vi "15_NOV_UPDATE_2.vi"() -> ()   [LabVIEW 2020]
uses:
  <instrlib>/Agilent B2900 Series/Agilent B2900 Series.lvlib
panel:
  out "Waveform Chart 2":dbl(graph)
  in  "Save data":bool
  in  "File_name":path=path "saved_data"
  out "Y -axis":string
  out "X -axis":string
  out "String":string
  out "SCPI Command":string
  out "?":bool
  in  "Time interval between iterations (seconds)":dbl
  out "?":cluster{"X":dbl[], "Y":dbl[]}[](graph)
  out "Waveform Chart":dbl(graph)
  out "Measured Output Value":dbl
  in  "SELECT DEVICE":refnum<visa-resource-name>="USB0::0x0957::0x8E18::MY51140695::INSTR"
  out "Resolution":dbl format="%#_6f"
  out "Instantaneous Input Value":dbl format="%#_6f"
  in  "Final Value":dbl
  in  "Initial Value":dbl
  in  "Steps":dbl
  in  "Measure (OUTPUT)":enum16{"Voltage", "Current"}(ring)
  in  "Source":enum16{"Voltage", "Current"}(ring)
  in  "Channel":u16(ring) items=["1", "2"]
  # "1. Include file extension .txt after filename while saving\n\n2. Give unique filename to avoid overwriting data."
  # "(INPUT)"
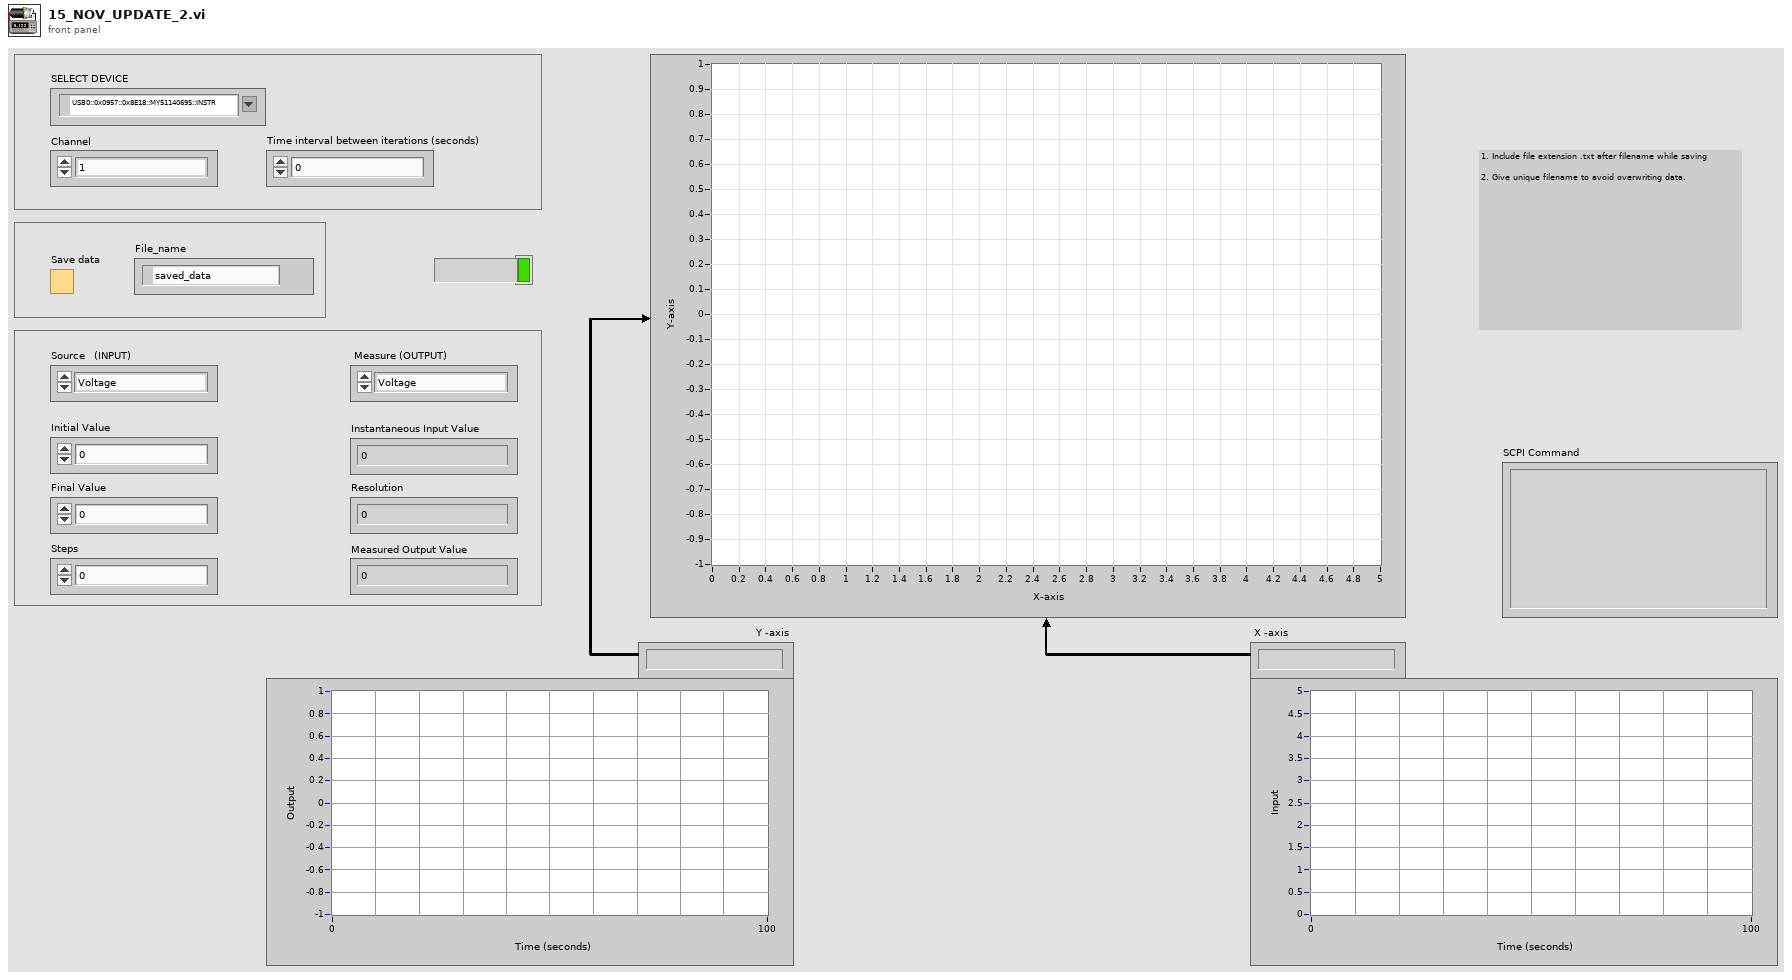
[diagram p1: front panel]
types:
  T1 = enum16{"open", "replace", "create", "open or create", "replace or create", "replace or create with confirmation"}
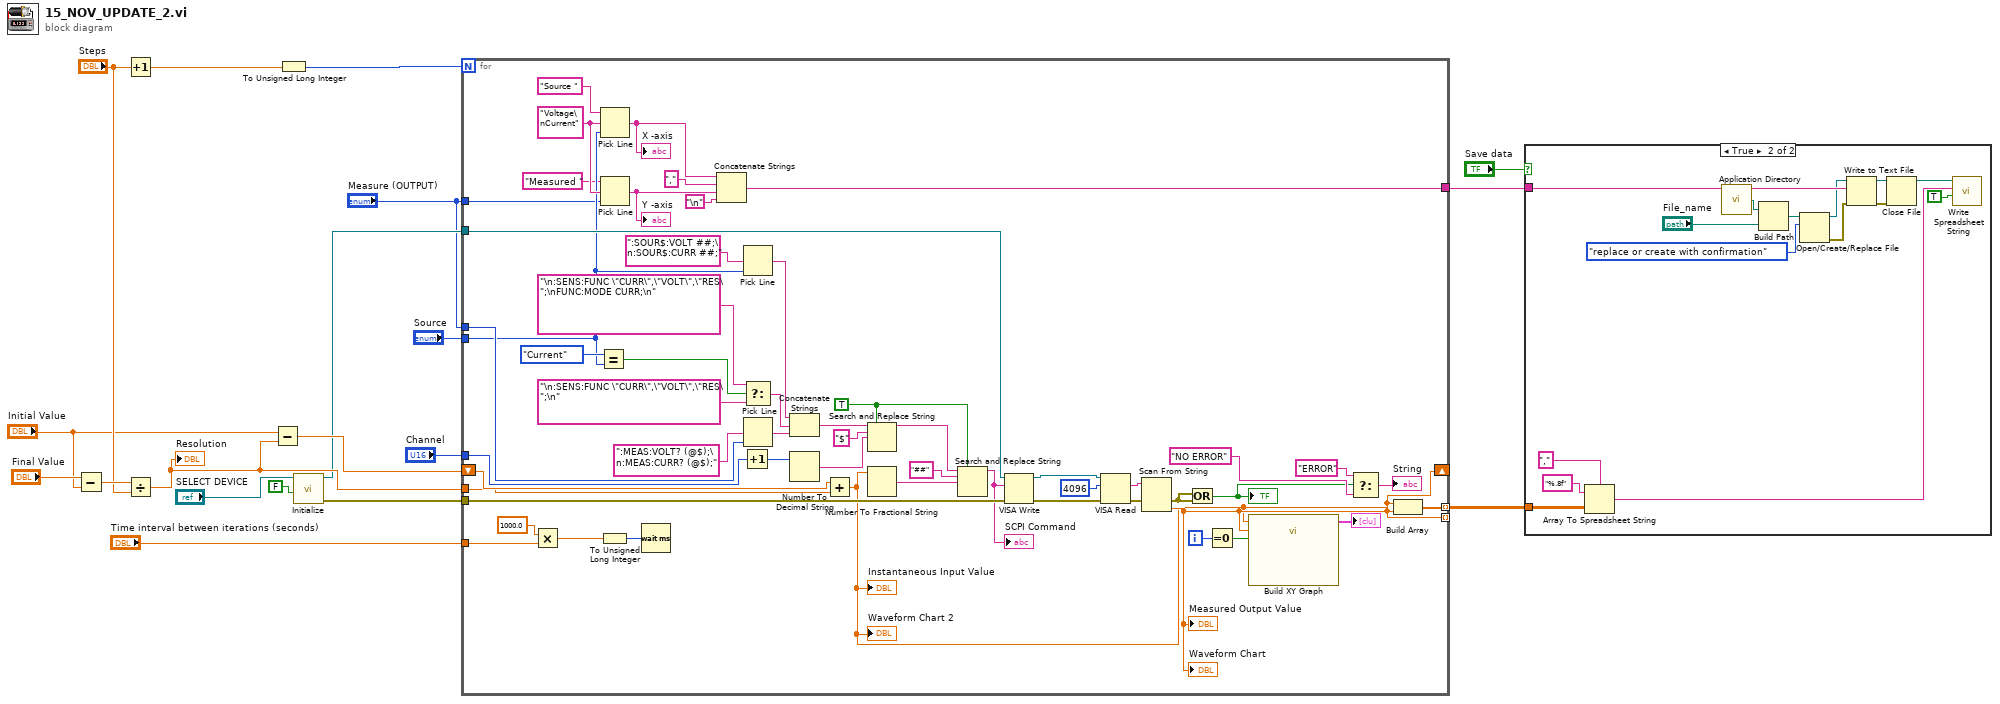
[diagram p0: block diagram]
diagram:
  n1 = Subtract(x="Final Value", y="Initial Value") -> (x-y=w15:dbl)
  n2 = Increment(x="Steps") -> (x+1=w6:dbl)
  n3 = Divide(x=w15, y="Steps") -> (x/y=w14:dbl)
  "Resolution" <- w14
  n4 = Subtract(x="Initial Value", y=w14) -> (x-y=w16:dbl)
  n5 = To Unsigned Long Integer(number=w6) -> (unsigned 32bit integer=w5:u32)
  n6 = call <instrlib>:"Initialize.vi"("Reset (True)"=FALSE, "VISA resource name"="SELECT DEVICE") -> ("error out"=w9:errorcluster, "VISA resource name out"=w10:refnum<visa-resource-name>)  [unwired: 8 in]
  n7 = for {
    N: w5 -> [_]
    tunnel: "Channel" -> [w72]
    tunnel: "Source" -> [w32]
    tunnel: "Measure (OUTPUT)" -> [w70]
    tunnel: w14 -> [w58]
    shift-right: [w25] -> _
    shift-left: w16 -> [w59]
    tunnel: w10 -> [w49]
    tunnel: w9 -> [w48]
    tunnel: "Time interval between iterations (seconds)" -> [w44]
    tunnel: "Measure (OUTPUT)" -> [w31]
    tunnel: [w27] -> _ mode=indexing
    tunnel: [w26] -> w2 mode=indexing
    tunnel: [w21] -> w1
    i -> [w46]
    w33 = "Voltage\nCurrent" ("multi-line string")
    w61 = TRUE ("replace all? (F)")
    n8 = Multiply(x=1000.0, y=w44) -> (x*y=w41:dbl)
    n9 = Equal?(x=enum16{"Voltage", "Current"}."Current", y=w32) -> (x = y?=w55:bool)
    n10 = To Unsigned Long Integer(number=w41) -> (unsigned 32bit integer=w42:u32)
    n11 = Pick Line(string ("")="Source ", multi-line string=w33, line index=w32) -> (output string=w24:string)
    "X -axis" <- w24
    n12 = Pick Line(string ("")="Measured ", multi-line string=w33, line index=w31) -> (output string=w23:string)
    "Y -axis" <- w23
    n13 = Wait (ms)(milliseconds to wait=w42) -> ()  [unwired: 1 out]
    n14 = Concatenate Strings(w24, "," ("string"), w23, "\n") -> (w21:string)
    n15 = Increment(x=w72) -> (x+1=w65:u16)
    n16 = Pick Line(multi-line string=":SOUR$:VOLT ##;\n:SOUR$:CURR ##;", line index=w32) -> (output string=w68:string)  [unwired: 1 in]
    n17 = Select(t="\n:SENS:FUNC \"CURR\",\"VOLT\",\"RES\";\nFUNC:MODE CURR;\n" ("string"), s=w55, f="\n:SENS:FUNC \"CURR\",\"VOLT\",\"RES\";\n") -> (s? t:f=w53:string)
    n18 = Pick Line(multi-line string=":MEAS:VOLT? (@$);\n:MEAS:CURR? (@$);", line index=w70) -> (output string=w69:string)  [unwired: 1 in]
    n19 = Concatenate Strings(w68, w53, w69) -> (w67:string)
    n20 = Number To Decimal String(number=w65) -> (decimal integer string=w64:string)  [unwired: 1 in]
    n21 = Add(x=w59, y=w58) -> (x+y=w25:dbl)
    "Instantaneous Input Value" <- w25
    "Waveform Chart 2" <- w25
    n22 = Search and Replace String(replace all?=w61, input string=w67, search string="$", replace string=w64) -> (result string=w63:string)  [unwired: 4 in, 3 out]
    n23 = Number To Fractional String(number=w25) -> (F-format string=w60:string)  [unwired: 3 in]
    n24 = Search and Replace String(replace all?=w61, input string=w63, search string="##", replace string=w60) -> (result string=w39:string)  [unwired: 4 in, 3 out]
    "SCPI Command" <- w39
    n25 = VISA Write(VISA resource name=w49, write buffer=w39, error in (no error)=w48) -> (VISA resource name out=w50:refnum<visa-resource-name>, error out=w51:errorcluster)  [unwired: 1 out]
    n26 = VISA Read(VISA resource name=w50, byte count=u32 4096, error in (no error)=w51) -> (read buffer=w47:string, error out=w38:errorcluster)  [unwired: 2 out]
    n27 = Scan From String(input string=w47, error in=w38) -> (error out=w40:errorcluster, output 1=w27:dbl)  [unwired: 3 in, 2 out]
    "Measured Output Value" <- w27
    "Waveform Chart" <- w27
    n28 = Or(x=w40, y=w40) -> (x .or. y?=w35:bool)
    "?" <- w35
    n29 = Equal To 0?(x=w46) -> (x = 0?=w45:bool)
    n30 = call "Build XY Graph"("Reset"=w45, "Y Input"=w27, "X Input"=w25) -> ("XY Graph"=→"?":cluster{"X":dbl[], "Y":dbl[]}[])  [unwired: 7 in, 1 out]
    n31 = Select(t="ERROR", s=w35, f="NO ERROR") -> (s? t:f=→"String":string)
    n32 = Build Array(w25, w27) -> (w26:dbl[])
  }
  n33 = case shown="True" "Save data" {
    tunnel: w2 -> [_ w79]
    tunnel: w1 -> [_ w78]
    frame False {
    }
    frame True {
      n34 = Array To Spreadsheet String(delimiter (Tab)=",", array=w79, 3:"%.8f" ("format string")) -> (spreadsheet string=w87:string)
      n35 = call <vilib>:"Application Directory.vi"() -> ("Application Directory"=w85:path)
      n36 = Build Path(base path=w85, name or relative path="File_name") -> (appended path=w83:path)
      n37 = Open/Create/Replace File(file path (use dialog)=w83, operation (0:open)=T1."replace or create with confirmation") -> (refnum out=w77:refnum<file>, error out=w76:errorcluster)  [unwired: 4 in, 1 out]
      n38 = Write to Text File(file (use dialog)=w77, text=w78, error in=w76) -> (refnum out=w75:refnum<file>, error out=w74:errorcluster)  [unwired: 1 in, 1 out]
      n39 = Close File(refnum=w75, error in=w74) -> (path=w82:path)  [unwired: 1 out]
      n40 = call <vilib>:"Write Spreadsheet String.vi"("append to file? (new file:F)"=TRUE, "spreadsheet string"=w87, "file path (dialog if empty)"=w82) -> ()  [unwired: 7 in, 2 out]
    }
  }
